vi "Install Octave Package golpi.vi"(6 "Verbose? (T)":bool=TRUE, 7 "feature":T1, 8 "error in":errorcluster, 10 "force reinstall? (F)":bool, 11 "GOLPI ref. in":T2={"pipe handle"={"lv_proc.dll file path"=path "", "process instance handle"=[], "debug mode"=FALSE, "debug data"=[]}, "fast read timeout [ms]"=500, "fast read settle time [ms]"=10, "fast read to multiple [ms]"=1, "max elements per input line"=100, "slow read timeout [ms]"=5000, "stdin double format specifier"="", "max elements per stdout output column"=100, "console mode bitstream"=FALSE, "bitstream first read timeout [ms]"=1000, "bitstream read timeout [ms]"=50, "struct transfer possible"=FALSE, "matlab mode"=FALSE, "var pipe write timeout [ms]"=5000, "variable pipe mode"=FALSE, "variable pipe buffer size [Bytes]"=10000000, "variable pipe block size [Bytes]"=1000000} {"variable pipe block size [Bytes]" format="%.0p"; "variable pipe buffer size [Bytes]" format="%.0p"}) -> (0 "error out":errorcluster, 3 "GOLPI ref. out":T2={"pipe handle"={"lv_proc.dll file path"=path "", "process instance handle"=[], "debug mode"=FALSE, "debug data"=[]}, "fast read timeout [ms]"=500, "fast read settle time [ms]"=10, "fast read to multiple [ms]"=1, "max elements per input line"=100, "slow read timeout [ms]"=5000, "stdin double format specifier"="", "max elements per stdout output column"=100, "console mode bitstream"=FALSE, "bitstream first read timeout [ms]"=1000, "bitstream read timeout [ms]"=50, "struct transfer possible"=FALSE, "matlab mode"=FALSE, "var pipe write timeout [ms]"=5000, "variable pipe mode"=FALSE, "variable pipe buffer size [Bytes]"=10000000, "variable pipe block size [Bytes]"=1000000} {"variable pipe block size [Bytes]" format="%.0p"; "variable pipe buffer size [Bytes]" format="%.0p"})   [LabVIEW 2020, in "GOLPI library.lvlib"]
doc: "Install GNU Octave package golpi. This package is required for Bitstream data transfer mode and for transfer of GNU Octave structures to LabVIEW clusters. VI search for package file golpi-X.X.X.tar.gz in application directory and subdirectories. If not found, a file dialog is opened for user to determine position of file. Input \"Feature name\" is used in description of message box. Input Verbose disables message box and file dialog.\n\n---\nGOLPI works only with lv_proc.dll library, which is part of vipm package or should be delivered together with packed library. Placement of this dll is selected in terminal of Start GNU Octave.vi."
uses:
  GOLPI library.lvlib
  Public/GOLPI reference Type Def.ctl
  LV Process source distribution/Pipe Handle.ctl
  Type Definitions/GOLPI package Feature.ctl
  Type Definitions/Custom Error Codes Enum Type Def.vi
  LV Process source distribution/LV Process library.lvlib
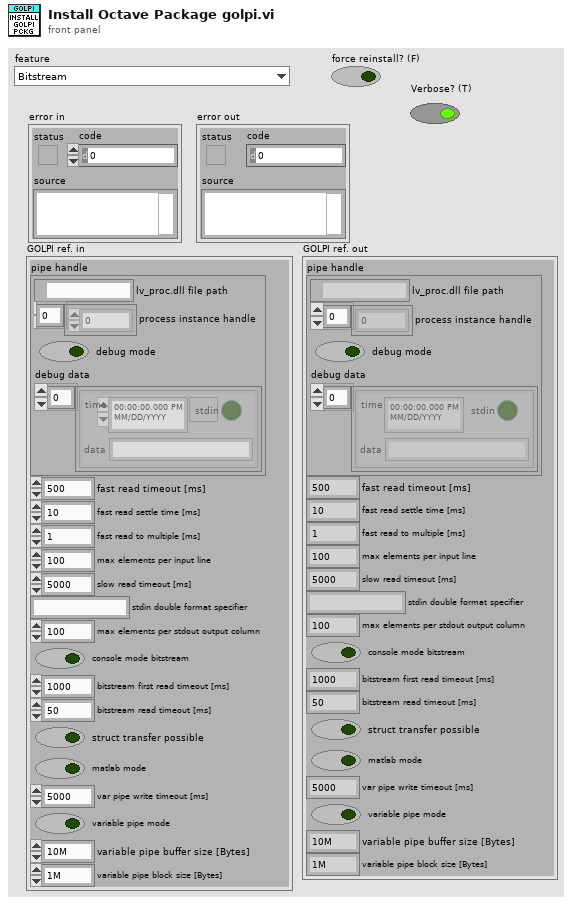
[diagram p1: front panel]
types:
  T1 = typedef "GOLPI package Feature.ctl" = enum16{"Bitstream", "Struct", "Pipes"}
  T2 = typedef "GOLPI library.lvlib/GOLPI reference Type Def.ctl" = cluster{"pipe handle":T3, "fast read timeout [ms]":u32, "fast read settle time [ms]":u32, "fast read to multiple [ms]":u32, "max elements per input line":u32, "slow read timeout [ms]":u32, "stdin double format specifier":string, "max elements per stdout output column":u32, "console mode bitstream":bool, "bitstream first read timeout [ms]":u32, "bitstream read timeout [ms]":u32, "struct transfer possible":bool, "matlab mode":bool, "var pipe write timeout [ms]":u32, "variable pipe mode":bool, "variable pipe buffer size [Bytes]":u32, "variable pipe block size [Bytes]":u32}
  T3 = typedef "LV Process library.lvlib/Pipe Handle.ctl" = cluster{"lv_proc.dll file path":path, "process instance handle":u32[], "debug mode":bool, "debug data":cluster{"time":timestamp, "stdin":bool, "data":string}[]}
  T4 = typedef "GOLPI library.lvlib/Custom Error Codes Enum Type Def.vi" = enum16{"no error", "00 working directory PAR1 missing", "01 octave binary PAR1 missing", "02 octave report error PAR1", "03 empty output last cmd PAR1", "04 missing temporary file PAR1", "05 pwd PAR 1 not exist", "06 oct package not installed", "07 octave default binary missing", "10 var PAR1 not string, vect", "11 var PAR1 not num, scal, ~compl", "12 var PAR1 not num, scal, compl", "13 var PAR1 not num, vect, ~compl", "14 var PAR1 not num, vect, compl", "15 var PAR1 not num, mat, ~compl", "16 var PAR1 not num, mat, ~compl", "30 read timeout", "60 bitstream transport failed", "61 bitstream decode error PAR1", "62 bitstream cannot be set", "70 struct transfer not possible", "80 struct: cluster elem. PAR1 not implem.", "81 struct: structure field PAR1 not implem.", "82 struct: size mismatch of PAR1", "83 struct: type mismatch of PAR1", "98 internal error", "99 not finished", "90 Not supported in Matlab mode", "91 Matlab variable transfer error", "92 Matlab Script Error", "100 Variable Pipe Mode cannot be set"}
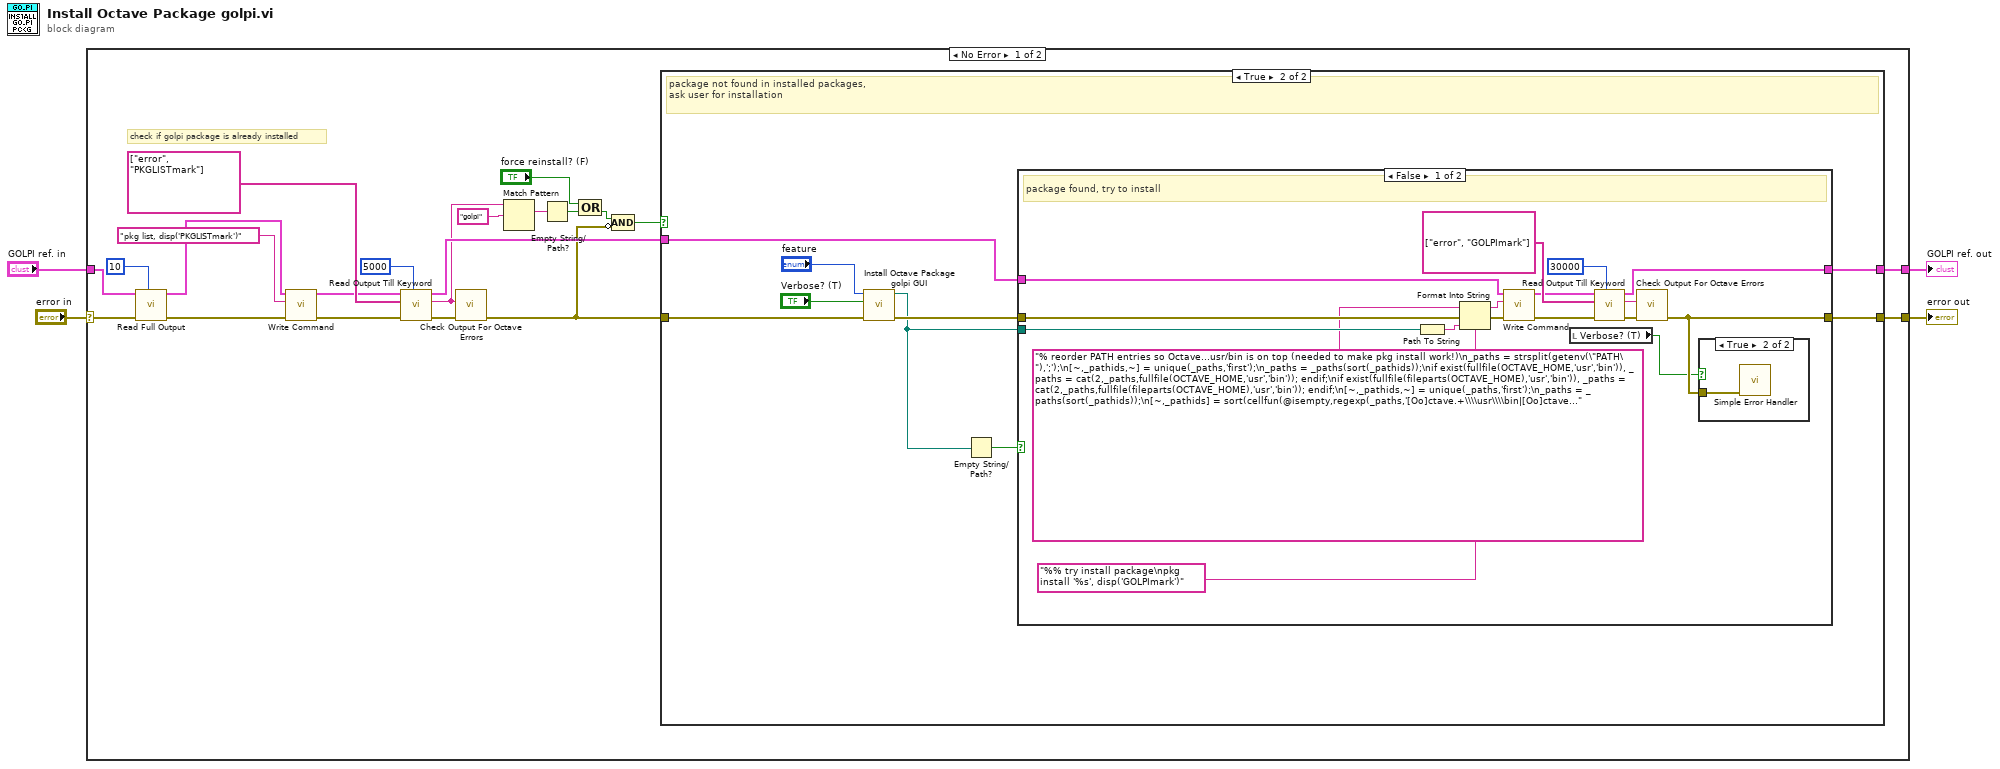
[diagram p0: block diagram]
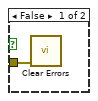
[diagram p3: hidden frame]
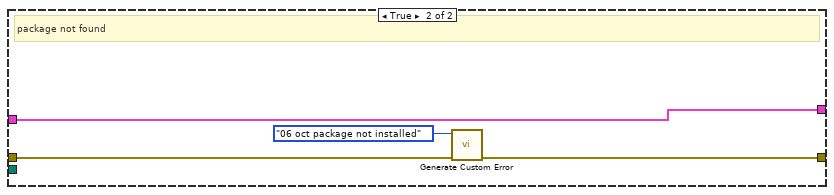
[diagram p4: hidden frame]
diagram:
  n1 = case shown="No Error" "error in" {
    selector: "error in" -> [w25 w62]
    tunnel: "GOLPI ref. in" -> [w26 w61]
    tunnel: [w13 w61] -> w3
    tunnel: [w24 w62] -> w1
    frame No Error {
      # "check if golpi package is already installed"
      n2 = call "Read Full Output.vi"("timeout [ms]"=u32 10, "error in"=w25, "GOLPI ref. in"=w26) -> ("error out"=w22:errorcluster, "GOLPI ref. out"=w23:T2)  [unwired: 5 in, 2 out]
      n3 = call "Write Command.vi"("error in"=w22, "command"="pkg list, disp('PKGLISTmark')", "GOLPI ref. in"=w23) -> ("error out"=w19:errorcluster, "GOLPI ref. out"=w18:T2)  [unwired: 7 in]
      n4 = call "Read Output Till Keyword.vi"("timeout [ms]"=u32 5000, "error in"=w19, "keywords"=string[] ["error", "PKGLISTmark"], "GOLPI ref. in"=w18) -> ("error out"=w10:errorcluster, "read buffer"=w9:string, "GOLPI ref. out"=w14:T2)  [unwired: 4 in, 1 out]
      n5 = call "Check Output For Octave Errors.vi"("error in"=w10, "read buffer"=w9) -> ("error out"=w8:errorcluster)  [unwired: 9 in]
      n6 = Match Pattern(string=w9, regular expression="golpi") -> (match substring=w11:string)  [unwired: 1 in, 3 out]
      n7 = Empty String/Path?(string/path=w11) -> (empty?=w6:bool)
      n8 = Compound Arithmetic op=OR("force reinstall? (F)", w6) -> (w7:bool)
      n9 = Compound Arithmetic op=AND(w7, invert w8) -> (w16:bool)
      n10 = case shown="True" w16 {
        tunnel: [w28 w37] -> w24
        tunnel: w8 -> [w28 w35]
        tunnel: w14 -> [w27 w31]
        tunnel: [w27 w36] -> w13
        frame False {
          # "package seems to be already installed,\nnothing to do"
        }
        frame True {
          # "package not found in installed packages,\nask user for installation"
          n11 = call "Install Octave Package golpi GUI.vi"("error in (no error)"=w35, "Verbose? (True)"="Verbose? (T)", "feature"="feature") -> ("error out"=w32:errorcluster, "Path"=w29:path)  [unwired: 7 in]
          n12 = Empty String/Path?(string/path=w29) -> (empty?=w30:bool)
          n13 = case shown="False" w30 {
            tunnel: w32 -> [w43 w58]
            tunnel: w31 -> [w48 w60]
            tunnel: w29 -> [w47 _]
            tunnel: [w40 w57] -> w37
            tunnel: [w41 w60] -> w36
            frame False {
              # "package found, try to install"
              n14 = Path To String(path=w47) -> (string=w45:string)
              n15 = Format Into String(format string="%% try install package\npkg install '%s', disp('GOLPImark')" ("command"), initial string="% reorder PATH entries so Octave...usr/bin is on top (needed to make pkg install work!)\n_paths = strsplit(getenv(\"PATH\"),';');\n[~,_pathids,~] = unique(_paths,'first');\n_paths = _paths(sort(_pathids));\nif exist(fullfile(OCTAVE_HOME,'usr','bin')), _paths = cat(2,_paths,fullfile(OCTAVE_HOME,'usr','bin')); endif;\nif exist(fullfile(fileparts(OCTAVE_HOME),'usr','bin')), _paths = cat(2,_paths,fullfile(fileparts(OCTAVE_HOME),'usr','bin')); endif;\n[~,_pathids,~] = unique(_paths,'first');\n_paths = _paths(sort(_pathids));\n[~,_pathids] = sort(cellfun(@isempty,regexp(_paths,'[Oo]ctave.+\\\\usr\\\\bin|[Oo]ctave.+\\\\bin')));\n_paths = _paths(_pathids);\nsetenv(\"PATH\",strjoin(_paths,';'));\nclear _paths _pathids;\n" ("command"), error in=w43, w45) -> (resulting string=w44:string, error out=w42:errorcluster)
              n16 = call "Write Command.vi"("error in"=w42, "command"=w44, "GOLPI ref. in"=w48) -> ("error out"=w53:errorcluster, "GOLPI ref. out"=w52:T2)  [unwired: 7 in]
              n17 = local read "Verbose? (T)"() -> (w38:bool)
              n18 = call "Read Output Till Keyword.vi"("timeout [ms]"=u32 30000, "error in"=w53, "keywords"=string[] ["error", "GOLPImark"], "GOLPI ref. in"=w52) -> ("error out"=w50:errorcluster, "read buffer"=w49:string, "GOLPI ref. out"=w41:T2)  [unwired: 4 in, 1 out]
              n19 = call "Check Output For Octave Errors.vi"("error in"=w50, "read buffer"=w49) -> ("error out"=w40:errorcluster)  [unwired: 9 in]
              n20 = case shown="True" w38 {
                tunnel: w40 -> [w55 w56]
                frame False {
                  n21 = call <vilib>:"Clear Errors.vi"("error in (no error)"=w55) -> ()  [unwired: 5 in, 2 out]
                }
                frame True {
                  n22 = call <vilib>:"Simple Error Handler.vi"("error in (no error)"=w56) -> ()  [unwired: 4 in, 5 out]
                }
              }
            }
            frame True {
              # "package not found"
              n23 = call "Generate Custom Error.vi"("error in"=w58, "GOLPI error"=Custom_Error_Codes_Enum_Type_Def.vi."06 oct package not installed") -> ("error out"=w57:errorcluster)  [unwired: 9 in]
            }
          }
        }
      }
    }
    frame Error {
    }
  }
  "error out" <- w1
  "GOLPI ref. out" <- w3
